vi "user_delete.vi"(7 "confirm deleting? (T)":bool=TRUE, 8 "error in (no error)":errorcluster, 10 "user name in":string) -> (0 "error out":errorcluster, 1 "cancelled?":bool)   [LabVIEW 2010]
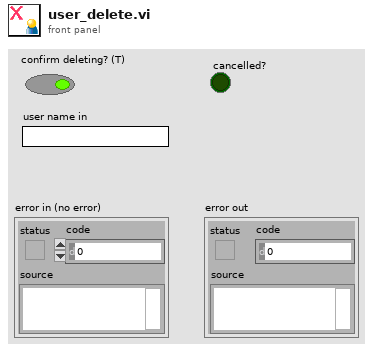
[diagram p1: front panel]
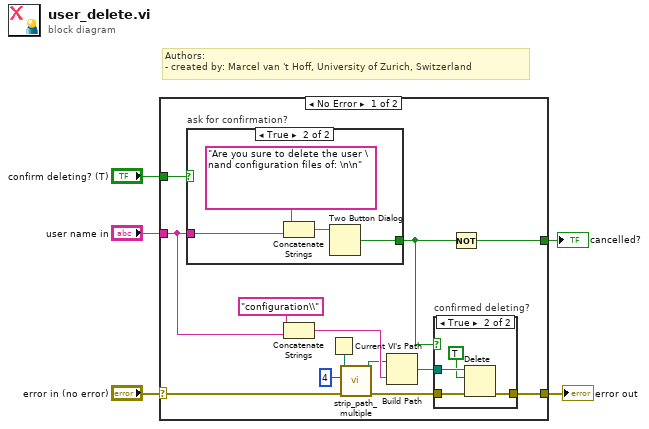
[diagram p0: block diagram]
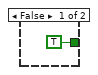
[diagram p2: hidden frame]
diagram:
  # "Authors: \n- created by: Marcel van 't Hoff, University of Zurich, Switzerland"
  n1 = case shown="No Error" "error in (no error)" {
    selector: "error in (no error)" -> [w10 w29]
    tunnel: [w11 w29] -> w5
    tunnel: "user name in" -> [w9 _]
    tunnel: "confirm deleting? (T)" -> [w8 _]
    tunnel: [w6 _] -> w1
    frame No Error {
      n2 = case "ask for confirmation?" shown="True" w8 {
        tunnel: [TRUE ("T button?") w21] -> w7
        tunnel: w9 -> [_ w20]
        frame False {
        }
        frame True {
          n3 = Concatenate Strings("Are you sure to delete the user \nand configuration files of: \n\n" ("message"), w20) -> (w22:string)
          n4 = Two Button Dialog(message=w22) -> (T button?=w21:bool)  [unwired: 2 in]
        }
      }
      n5 = Concatenate Strings("configuration\\" ("name or relative path"), w9) -> (w15:string)
      n6 = Current VI's Path() -> (path=w18:path)
      n7 = call "strip_path_multiple.vi"("error in (no error)"=w10, "number of strips"=4, "path in"=w18) -> ("error out"=w12:errorcluster, "path out"=w14:path)  [unwired: 7 in]
      n8 = Build Path(base path=w14, name or relative path=w15) -> (appended path=w13:path)
      n9 = case "confirmed deleting?" shown="True" w7 {
        tunnel: w13 -> [_ w28]
        tunnel: w12 -> [w24 w27]
        tunnel: [w24 w25] -> w11
        frame False {
        }
        frame True {
          n10 = Delete(path (use dialog)=w28, entire hierarchy (F)=TRUE, error in=w27) -> (error out=w25:errorcluster)  [unwired: 2 in, 2 out]
        }
      }
      n11 = Not(x=w7) -> (.not. x?=w6:bool)
    }
    frame Error {
    }
  }
  "error out" <- w5
  "cancelled?" <- w1
